vi "XYZ MovePause.vi"(3 "Notify?":bool=TRUE, 4 "Refnums":T2, 5 "Notifications":T1, 6 "Wait For Motion Done?":bool, 7 "Instrument Status":refnum<vi>, 8 "error in (no error)":errorcluster, 9 "Motion Mode":enum16{"Absolute", "Relative"}(ring), 10 "Destination [mm]":dbl[](array[numeric])=[-4692.2, 3210.5, -4992.395238095239], 11 "LSID":i32=1) -> (0 "error out":errorcluster, 2 "Position":dbl[](array[numeric])=[-4692.2, 3210.5, -4992.4])   [LabVIEW 2014]
uses:
  XYZ Refnums.ctl
  support/Instrument Status.ctl
  XYZ Stage Control.ctl
  <instrlib>/Tango Drivers/Labview/SubVIs/Axis_Switch.ctl
  XYZ Notifications.ctl
  support/Instrument Status State.ctl
panel:
  in  "Stop here if it hangs":bool
  # "LICENSED MATERIALS – PROPERTY OF IBM\nCopyright IBM Corp. 2016,\nALL RIGHTS RESERVED"
  # "XY"
  # "Z"
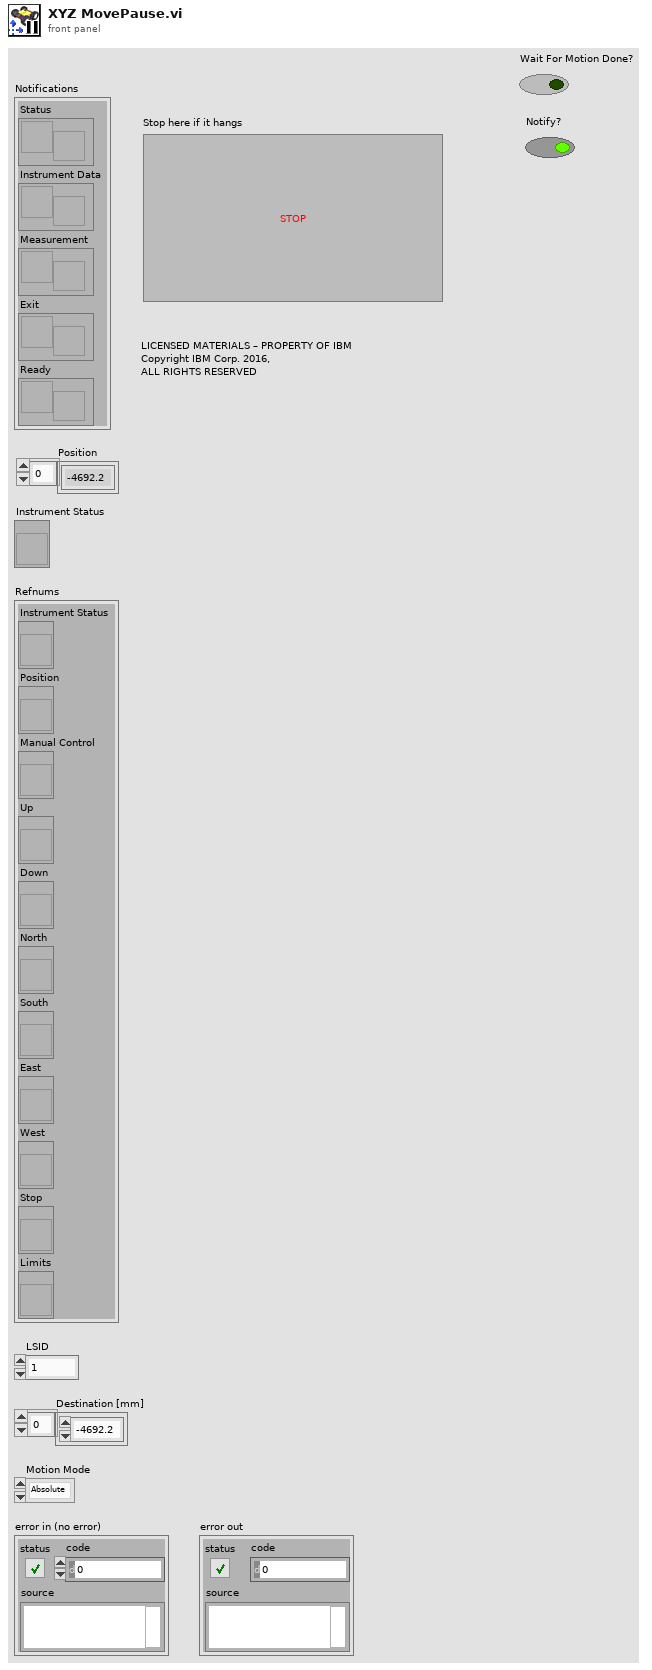
[diagram p1: front panel]
types:
  T1 = typedef "XYZ Notifications.ctl" = cluster{"Status":refnum<notifier>, "Instrument Data":refnum<notifier>, "Measurement":refnum<notifier>, "Exit":refnum<notifier>, "Ready":refnum<notifier>}
  T2 = typedef "XYZ Refnums.ctl" = cluster{"Instrument Status":refnum<vi>, "Position":refnum<vi>, "Manual Control":refnum<vi>, "Up":refnum<vi>, "Down":refnum<vi>, "North":refnum<vi>, "South":refnum<vi>, "East":refnum<vi>, "West":refnum<vi>, "Stop":refnum<vi>, "Limits":refnum<vi>}
  T3 = typedef "Instrument Status State.ctl" = enum16{"Unknown", "Idle", "Standby", "Configuring", "Measuring", "Moving", "Disconnected"}
  T4 = enum16{"Axis Stand Still", "Axis in Motion", "Axis Disabled", "Joystick on", "Axis in Closed Loop", "Return Message After Calibration", "Calibration Error", "Return Message after Travel", "Setup Mode", "Timeout", "Status Unknown"}[]
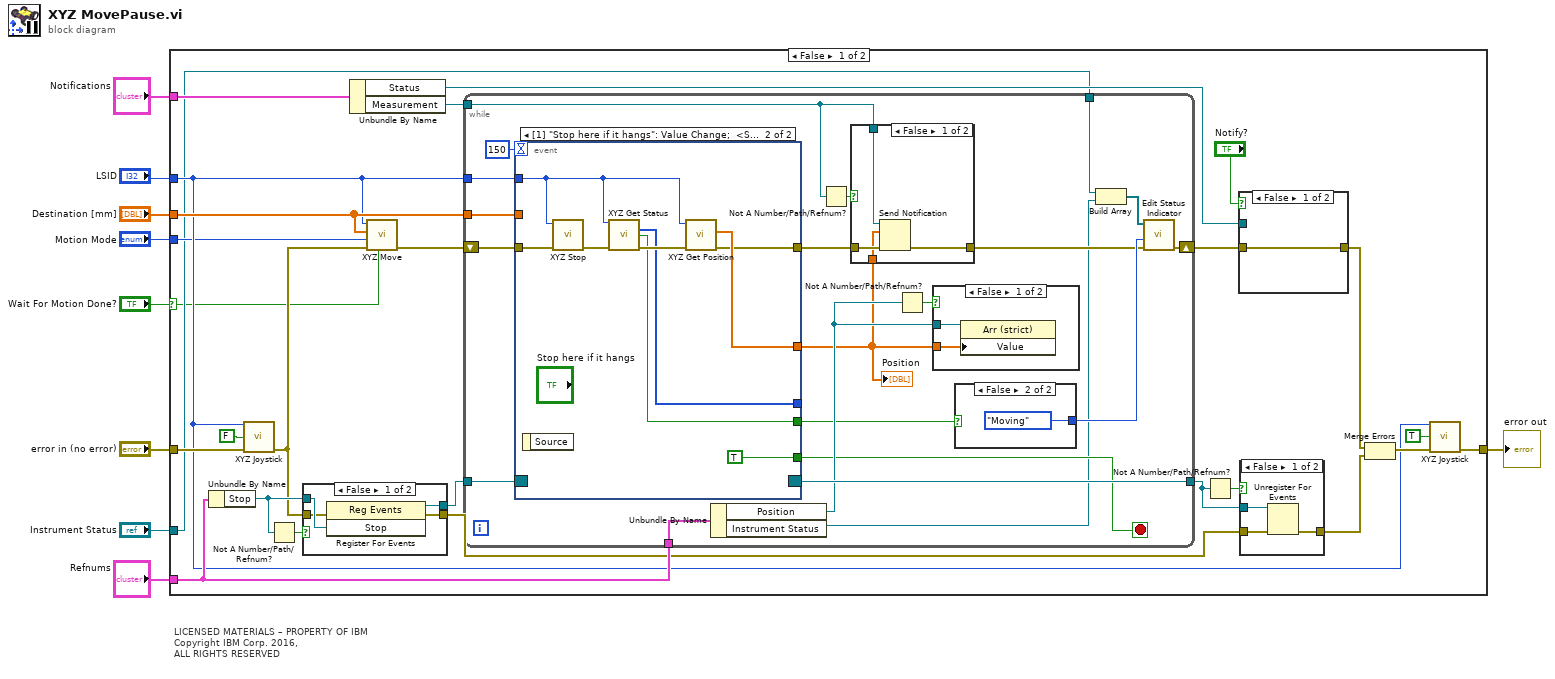
[diagram p0: block diagram]
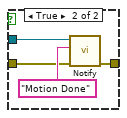
[diagram p2: hidden frame]
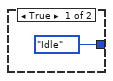
[diagram p3: hidden frame]
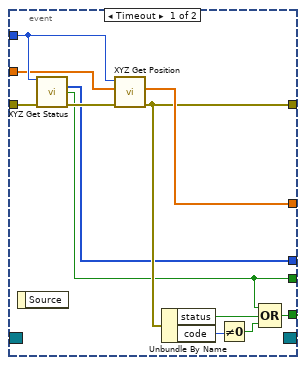
[diagram p5: hidden frame]
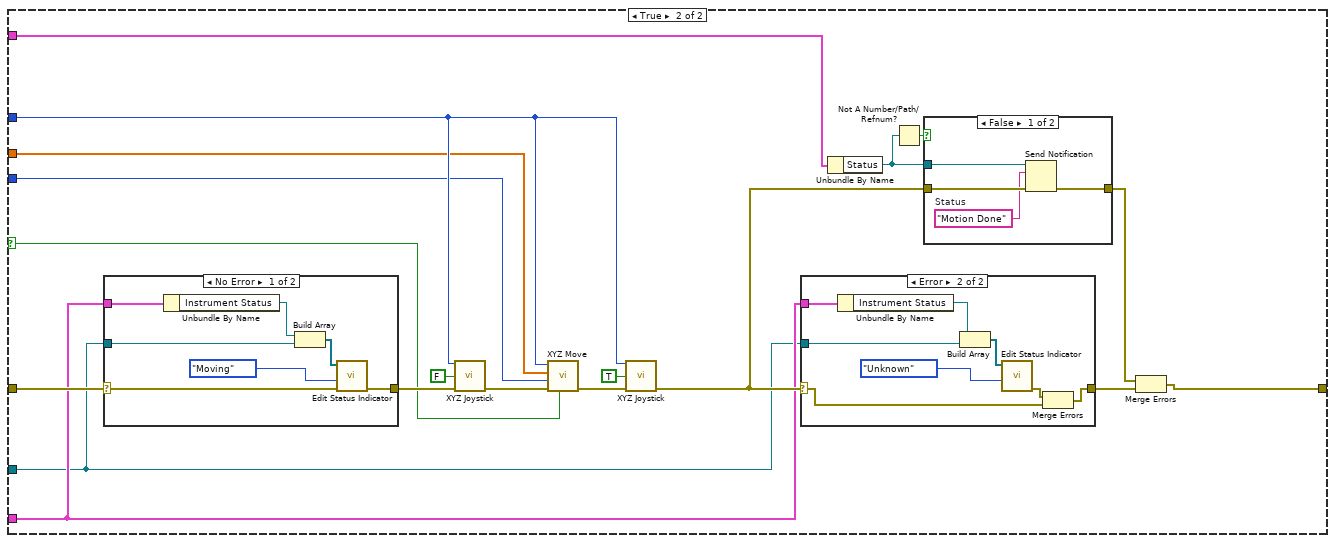
[diagram p9: hidden frame]
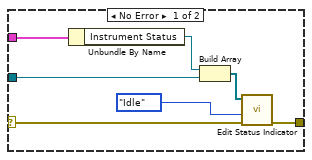
[diagram p11: hidden frame]
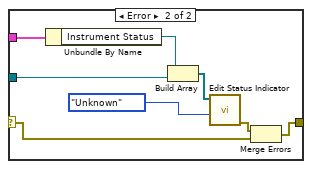
[diagram p12: hidden frame]
diagram:
  # "LICENSED MATERIALS – PROPERTY OF IBM\nCopyright IBM Corp. 2016,\nALL RIGHTS RESERVED"
  n1 = case shown="False" "Wait For Motion Done?" {
    selector: "Wait For Motion Done?" -> [w11 w101]
    tunnel: "Notifications" -> [w35 w109]
    tunnel: "LSID" -> [w14 w107]
    tunnel: "Refnums" -> [w34 w105]
    tunnel: [w15 w104] -> w5
    tunnel: "error in (no error)" -> [w19 w108]
    tunnel: "Destination [mm]" -> [w33 w106]
    tunnel: "Motion Mode" -> [w13 w103]
    tunnel: "Instrument Status" -> [w12 w102]
    frame False {
      n2 = Unbundle By Name(w34) -> ("Stop"=w29:refnum<vi>)
      n3 = call "XYZ Joystick.vi"("LSID"=w14, "Joystick on?"=FALSE, "error in (no error)"=w19) -> ("error out"=w18:errorcluster)  [unwired: 12 in]
      n4 = Not A Number/Path/Refnum?(number/path/refnum=w29) -> (NaN/Path/Refnum?=w31:bool)
      n5 = case shown="False" w31 {
        tunnel: w29 -> [w99 _]
        tunnel: [w98 _] -> w26
        tunnel: [w97 w100] -> w28
        tunnel: w18 -> [w96 w100]
        frame False {
          n6 = register-events(error in=w96, w99) -> (reference out=w98:refnum<event-registration>, error out=w97:errorcluster)  [unwired: 1 in]
        }
        frame True {
        }
      }
      n7 = Unbundle By Name(w35) -> ("Status"=w21:refnum<notifier>, "Measurement"=w24:refnum<notifier>)
      n8 = call "XYZ Move.vi"("Wait For Motion Done?"=w11, "error in (no error)"=w18, "Motion Mode"=w13, "Destination [mm]"=w33, "LSID"=w14) -> ("error out"=w32:errorcluster)  [unwired: 6 in]
      n9 = while "Polling until the destination is reached or Error occurs" {
        tunnel: w26 -> [w57]
        tunnel: [w56] -> w25
        tunnel: w34 -> [w58]
        tunnel: w24 -> [w52]
        shift-right: [w47] -> w23
        shift-left: w32 -> [w61]
        tunnel: w14 -> [w44]
        tunnel: w33 -> [w43]
        tunnel: w12 -> [w41]
        stop <- w53 stop-if-true
        n10 = event shown="[1] \"Stop here if it hangs\": Value Change;  <Stop>: Value Change" {
          selector: w57 -> [_ _]
          dyn-events: [_ _] -> w56
          timeout: 150 -> [_ _]
          tunnel: [w75 w86] -> w59
          tunnel: [w76 w88] -> w45
          tunnel: [w77 TRUE] -> w53
          tunnel: [w69 w81] -> w42
          tunnel: w61 -> [w74 w87]
          tunnel: w44 -> [w72 w83]
          tunnel: w43 -> [w71 _]
          tunnel: [w70 w82] -> _
          event Timeout {
            n11 = event-data() -> ()  [unwired: 2 out]
            n12 = call "XYZ Get Status.vi"("LSID in"=w72, "error in (no error)"=w74) -> ("Axis Status"=w70:T4, "Motion Done?"=w69:bool, "error out"=w73:errorcluster)  [unwired: 9 in, 2 out]
            n13 = call "XYZ Get Position.vi"("error in (no error)"=w73, "Pos In in"=w71, "LSID"=w72) -> ("error out"=w75:errorcluster, "Pos In out"=w76:dbl[])  [unwired: 7 in]
            n14 = Unbundle By Name(w75) -> ("status"=w79:bool, "code"=w80:i32)
            n15 = Not Equal To 0?(x=w80) -> (x != 0?=w78:bool)
            n16 = Compound Arithmetic op=OR(w69, w79, w78) -> (w77:bool)
          }
          event "Stop here if it hangs": Value Change {
            n17 = event-data() -> ()  [unwired: 2 out]
            n18 = call "XYZ Stop.vi"("error in (no error)"=w87, "LSID"=w83) -> ("error out"=w85:errorcluster)  [unwired: 9 in]
            n19 = call "XYZ Get Status.vi"("LSID in"=w83, "error in (no error)"=w85) -> ("Axis Status"=w82:T4, "Motion Done?"=w81:bool, "error out"=w84:errorcluster)  [unwired: 9 in, 2 out]
            n20 = call "XYZ Get Position.vi"("error in (no error)"=w84, "LSID"=w83) -> ("error out"=w86:errorcluster, "Pos In out"=w88:dbl[])  [unwired: 8 in]
          }
        }
        "Position" <- w45
        n21 = Unbundle By Name(w58) -> ("Position"=w54:refnum<vi>, "Instrument Status"=w46:refnum<vi>)
        n22 = Not A Number/Path/Refnum?(number/path/refnum=w52) -> (NaN/Path/Refnum?=w51:bool)
        n23 = case shown="False" w51 {
          tunnel: w59 -> [w67 w68]
          tunnel: [w66 w68] -> w48
          tunnel: w52 -> [w65 _]
          tunnel: w45 -> [w64 _]
          frame False {
            n24 = Send Notification(notification=w64, notifier=w65, error in (no error)=w67) -> (error out=w66:errorcluster)  [unwired: 1 out]
          }
          frame True {
          }
        }
        n25 = Not A Number/Path/Refnum?(number/path/refnum=w54) -> (NaN/Path/Refnum?=w55:bool)
        n26 = case shown="False" w55 {
          tunnel: w45 -> [w90 _]
          tunnel: w54 -> [w91 _]
          frame False {
            n27 = property class="Arr (strict)"(reference=w91, "Value"=w90) -> ()  [unwired: 1 in, 2 out]
          }
          frame True {
          }
        }
        n28 = case shown="False" w42 {
          tunnel: [Instrument_Status_State."Idle" ("State") Instrument_Status_State."Moving" ("State")] -> w50
          frame True {
          }
          frame False {
          }
        }
        n29 = Build Array(w41, w46) -> (w49:refnum<vi>[])
        n30 = call "Edit Status Indicator.vi"("error in (no error)"=w48, "State"=w50, "Instrument Status Refnum"=w49) -> ("error out"=w47:errorcluster)  [unwired: 1 in, 7 out]
      }
      n31 = Not A Number/Path/Refnum?(number/path/refnum=w25) -> (NaN/Path/Refnum?=w30:bool)
      n32 = case shown="False" "Notify?" {
        tunnel: w23 -> [w36 w38]
        tunnel: [w36 w37] -> w22
        tunnel: w21 -> [_ w39]
        frame False {
        }
        frame True {
          n33 = call "Notify.vi"("error in (no error)"=w38, "String"="Motion Done", "Notifier in"=w39) -> ("error out"=w37:errorcluster)  [unwired: 8 in]
        }
      }
      n34 = case shown="False" w30 {
        tunnel: w28 -> [w94 w95]
        tunnel: [w93 w95] -> w27
        tunnel: w25 -> [w92 _]
        frame False {
          n35 = Unregister For Events(event registration refnum=w92, error in=w94) -> (error out=w93:errorcluster)
        }
        frame True {
        }
      }
      n36 = Merge Errors(w22, w27) -> (w16:errorcluster)
      n37 = call "XYZ Joystick.vi"("LSID"=w14, "Joystick on?"=TRUE, "error in (no error)"=w16) -> ("error out"=w15:errorcluster)  [unwired: 12 in]
    }
    frame True {
      n38 = case shown="No Error" w108 {
        selector: w108 -> [w145 w152]
        tunnel: [w144 w151] -> w114
        tunnel: w105 -> [w141 w148]
        tunnel: w102 -> [w140 w147]
        frame No Error {
          n39 = Unbundle By Name(w141) -> ("Instrument Status"=w142:refnum<vi>)
          n40 = Build Array(w142, w140) -> (w143:refnum<vi>[])
          n41 = call "Edit Status Indicator.vi"("error in (no error)"=w145, "State"=Instrument_Status_State."Moving", "Instrument Status Refnum"=w143) -> ("error out"=w144:errorcluster)  [unwired: 1 in, 7 out]
        }
        frame Error {
          n42 = Unbundle By Name(w148) -> ("Instrument Status"=w149:refnum<vi>)
          n43 = Build Array(w149, w147) -> (w153:refnum<vi>[])
          n44 = call "Edit Status Indicator.vi"("State"=Instrument_Status_State."Unknown", "Instrument Status Refnum"=w153) -> ("error out"=w150:errorcluster)  [unwired: 2 in, 7 out]
          n45 = Merge Errors(w150, w152) -> (w151:errorcluster)
        }
      }
      n46 = call "XYZ Joystick.vi"("LSID"=w107, "Joystick on?"=FALSE, "error in (no error)"=w114) -> ("error out"=w113:errorcluster)  [unwired: 12 in]
      n47 = call "XYZ Move.vi"("Wait For Motion Done?"=w101, "error in (no error)"=w113, "Motion Mode"=w103, "Destination [mm]"=w106, "LSID"=w107) -> ("error out"=w111:errorcluster)  [unwired: 6 in]
      n48 = call "XYZ Joystick.vi"("LSID"=w107, "Joystick on?"=TRUE, "error in (no error)"=w111) -> ("error out"=w110:errorcluster)  [unwired: 12 in]
      n49 = case shown="Error" w110 {
        selector: w110 -> [w130 w137]
        tunnel: [w129 w136] -> w116
        tunnel: w105 -> [w126 w133]
        tunnel: w102 -> [w125 w132]
        frame No Error {
          n50 = Unbundle By Name(w126) -> ("Instrument Status"=w127:refnum<vi>)
          n51 = Build Array(w127, w125) -> (w128:refnum<vi>[])
          n52 = call "Edit Status Indicator.vi"("error in (no error)"=w130, "State"=Instrument_Status_State."Idle", "Instrument Status Refnum"=w128) -> ("error out"=w129:errorcluster)  [unwired: 1 in, 7 out]
        }
        frame Error {
          n53 = Unbundle By Name(w133) -> ("Instrument Status"=w134:refnum<vi>)
          n54 = Build Array(w134, w132) -> (w138:refnum<vi>[])
          n55 = call "Edit Status Indicator.vi"("State"=Instrument_Status_State."Unknown", "Instrument Status Refnum"=w138) -> ("error out"=w135:errorcluster)  [unwired: 2 in, 7 out]
          n56 = Merge Errors(w135, w137) -> (w136:errorcluster)
        }
      }
      n57 = Unbundle By Name(w109) -> ("Status"=w117:refnum<notifier>)
      n58 = Not A Number/Path/Refnum?(number/path/refnum=w117) -> (NaN/Path/Refnum?=w118:bool)
      n59 = case shown="False" w118 {
        tunnel: w117 -> [w123 _]
        tunnel: w110 -> [w122 w124]
        tunnel: [w121 w124] -> w119
        frame False {
          w120 = "Motion Done"  # Status
          n60 = Send Notification(notification=w120, notifier=w123, error in (no error)=w122) -> (error out=w121:errorcluster)  [unwired: 1 out]
        }
        frame True {
        }
      }
      n61 = Merge Errors(w119, w116) -> (w104:errorcluster)
    }
  }
  "error out" <- w5
